vi "StartNewFile.vi"(8 "error in (no error)":errorcluster, 9 "Root File Name":string, 10 "Data Files Folder Path":path, 11 "DataLogRaster in":refnum<class "DataLogRaster.lvclass">) -> (0 "error out":errorcluster, 3 "DataLogRaster out":refnum<class "DataLogRaster.lvclass">)   [LabVIEW 2019, in "DataLogRaster.lvclass"]
doc: "Create absolute file path for the test sequence.\nGive it a date and time tag so it is always unique (for now)."
uses:
  DataLogRaster.lvclass
  DataLogRaster.lvclass/DataLogRaster.ctl
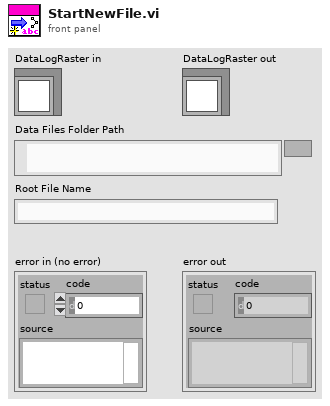
[diagram p1: front panel]
types:
  T1 = enum16{"open", "replace", "create", "open or create", "replace or create", "replace or create with confirmation"}
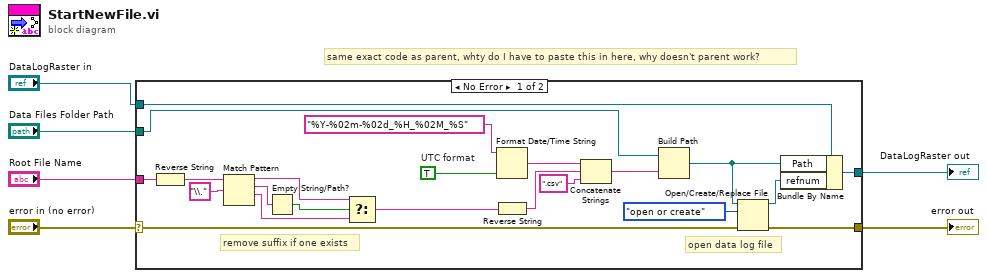
[diagram p0: block diagram]
diagram:
  # "same exact code as parent, whty do I have to paste this in here, why doesn't parent work?"
  n1 = case shown="No Error" "error in (no error)" {
    selector: "error in (no error)" -> [w9 w30]
    tunnel: [w8 w30] -> w4
    tunnel: [w13 w29] -> w5
    tunnel: "DataLogRaster in" -> [w14 w29]
    tunnel: "Root File Name" -> [w21 _]
    tunnel: "Data Files Folder Path" -> [w15 _]
    frame No Error {
      w7 = TRUE  # UTC format
      # "open data log file"
      # "remove suffix if one exists"
      n2 = Reverse String(1:w21) -> (0:w22:string)
      n3 = Match Pattern(string=w22, regular expression="\\.") -> (before substring=w24:string, match substring=w25:string, after substring=w28:string)  [unwired: 1 in, 1 out]
      n4 = Empty String/Path?(string/path=w25) -> (empty?=w27:bool)
      n5 = Select(t=w24, s=w27, f=w28) -> (s? t:f=w26:string)
      n6 = Format Date/Time String(time format string (%c)="%Y-%02m-%02d_%H_%02M_%S", UTC format=w7) -> (date/time string=w19:string)  [unwired: 1 in]
      n7 = Reverse String(1:w26) -> (0:w18:string)
      n8 = Concatenate Strings(w19, w18, ".csv" ("string")) -> (w16:string)
      n9 = Build Path(base path=w15, name or relative path=w16) -> (appended path=w10:path)
      n10 = Open/Create/Replace File(file path (use dialog)=w10, error in=w9, operation (0:open)=T1."open or create") -> (refnum out=w11:refnum<file>, error out=w8:errorcluster)  [unwired: 3 in, 1 out]
      n11 = Bundle By Name(cluster=w14, "Path"=w10, "refnum"=w11) -> (w13:refnum<class "DataLogRaster.lvclass">)
    }
    frame Error {
    }
  }
  "error out" <- w4
  "DataLogRaster out" <- w5
